vi "Erosion.vi"() -> ()   [LabVIEW 2018]
doc: "Erosion: This example is an example of image corrosion processing. This example is used for morphological image processing in image processing. It is mainly used to reduce the boundaries of objects in images or remove small noise, in order to better extract targets or perform subsequent analysis. In the corrosion operation, each pixel in the image is considered as an element of a set, which is composed of neighborhoods around the pixels. For each pixel, the corrosion operation sets its value to the minimum value in the neighborhood."
uses:
  vi.lib/VIRobotics/opencv_yiku/Mat/Mat_8U/Mat_8U.lvclass
  D:/Program Files/company/National Instruments/LabVIEW 2018/vi.lib/addons/VIRobotics/opencv_yiku/Mat/Mat/Mat.lvclass
  vi.lib/VIRobotics/opencv_yiku/Mat/Create_Mat_8U.vi
  vi.lib/VIRobotics/opencv_yiku/opencv_yiku.lvlib
panel:
  out "picture":picture
  in  "shape":T1(ring)
  in  "size":cluster{"x":i32, "y":i32}={"x"=3, "y"=3}
  out "erode picture":picture
  # "Overview: The basic idea of erosion is just like soil erosion only, it erodes away the boundaries of foreground object (Always try to keep foreground in white). So what it does? The kernel slides through the image (as in 2D convolution). A pixel in the original image (either 1 or 0) will be considered 1 only if all the pixels under the kernel is 1, otherwise it is eroded (made to zero).So what happends is that, all the pixels near boundary will be discarded depending upon the size of kernel. So the thickness or size of the foreground object decreases or simply white region decreases in the image. It is useful for removing small white noises (as we have seen in colorspace chapter), detach two connected objects etc.\nRequirements: Windows.\nInstructions: \n1.Run the VI"
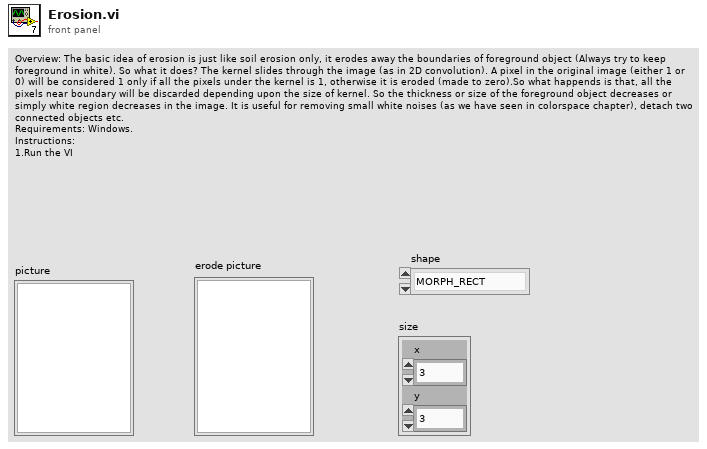
[diagram p1: front panel]
types:
  T1 = enum16{"MORPH_RECT", "MORPH_CROSS", "MORPH_ELLIPSE"}
  T2 = enum32{"COLOR_BGR2BGRA", "COLOR_BGRA2BGR", "COLOR_BGR2RGBA", "COLOR_RGBA2BGR", "COLOR_BGR2RGB", "COLOR_BGRA2RGBA", "COLOR_BGR2GRAY", "COLOR_RGB2GRAY", "COLOR_GRAY2BGR", "COLOR_GRAY2BGRA"}
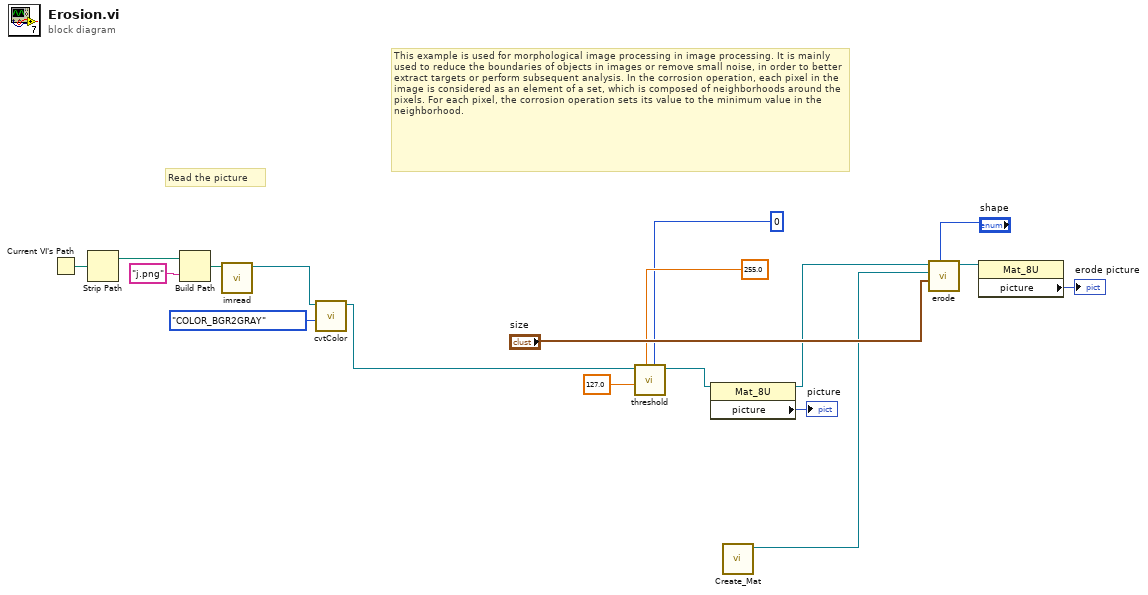
[diagram p0: block diagram]
diagram:
  # "This example is used for morphological image processing in image processing. It is mainly used to reduce the boundaries of objects in images or remove small noise, in order to better extract targets or perform subsequent analysis. In the corrosion operation, each pixel in the image is considered as an element of a set, which is composed of neighborhoods around the pixels. For each pixel, the corrosion operation sets its value to the minimum value in the neighborhood."
  # "Read the picture"
  n1 = Current VI's Path() -> (path=w17:path)
  n2 = Strip Path(path=w17) -> (stripped path=w18:path)  [unwired: 1 out]
  n3 = Build Path(base path=w18, name or relative path="j.png") -> (appended path=w15:path)
  n4 = call "imread.vi"("path"=w15) -> ("Mat out"=w10:refnum<class "Mat_8U.lvclass">)  [unwired: 9 in, 1 out]
  n5 = call "cvtColor.vi"("dstCn"=T2."COLOR_BGR2GRAY", "src"=w10) -> ("src out"=w5:refnum<class "Mat_8U.lvclass">)  [unwired: 7 in, 2 out]
  n6 = call "threshold.vi"("type"=0, "maxval"=255.0, "thresh"=127.0, "Mat in"=w5) -> ("dst out"=w3:refnum<class "Mat_8U.lvclass">)  [unwired: 6 in, 1 out]
  n7 = property class="Mat_8U"(reference=w3) -> (reference out=w2:refnum<class "Mat_8U.lvclass">, "picture"=→"picture":picture)  [unwired: 1 in, 1 out]
  n8 = call-poly "Create_Mat.vi"() -> ("Mat_8U_out"=w1:refnum<class "Mat_8U.lvclass">)  [unwired: 10 in, 1 out]
  n9 = call "erode.vi"("shape"="shape", "size"="size", "dst in"=w1, "Mat in"=w2) -> ("dst out"=w13:refnum<class "Mat_8U.lvclass">)  [unwired: 6 in, 1 out]
  n10 = property class="Mat_8U"(reference=w13) -> ("picture"=→"erode picture":picture)  [unwired: 1 in, 2 out]
